vi "PH_Get6PInformation.set Sixpack Configuration.vi"(1 "Motor Type":T1, 2 "6P Axis Config Ref":refnum<vi>) -> (0 "6P Axis Config":T2 {"Axis Parameter"."Poslimit (6400)" step=1; "Ref Search Parameter"."DebouncingTime (22ms)" format="%.0x"; "I max (50%)" min=0.0 max=100.0})   [LabVIEW 2014, in "PH_Get6PInformation.lvlib"]
uses:
  PH_Get6PInformation.lvlib
  PH_Sixpack/PH_Sixpack.Axis Configuration.ctl
  instr.lib/SixPack/PackDLL/VmaxAmax.ctl
  instr.lib/SixPack/PackDLL/PeakCurrent.ctl
  instr.lib/SixPack/PackDLL/VStartVmin.ctl
  instr.lib/SixPack/PackDLL/Ref Search Parameter.ctl
  instr.lib/SixPack/PackDLL/Stopswitch Limits.ctl
  instr.lib/SixPack/PackDLL/Motor Parameter.ctl
  instr.lib/SixPack/PackDLL/MotorParameter_P5.ctl
  instr.lib/SixPack/PackDLL/MotorParameter_P6.ctl
  instr.lib/SixPack/PackDLL/Current Control.ctl
  instr.lib/SixPack/PackDLL/Current.ctl
  PH_Stepmotor_BaseClass/PH_Stepmotor_BaseClass.Motor Type.ctl
  PH_Sixpack/PH_Sixpack.lvlib
  instr.lib/SixPack/Sixpack - Driver.lvlib
  PH_Stepmotor_BaseClass/PH_Stepmotor_BaseClass.lvlib
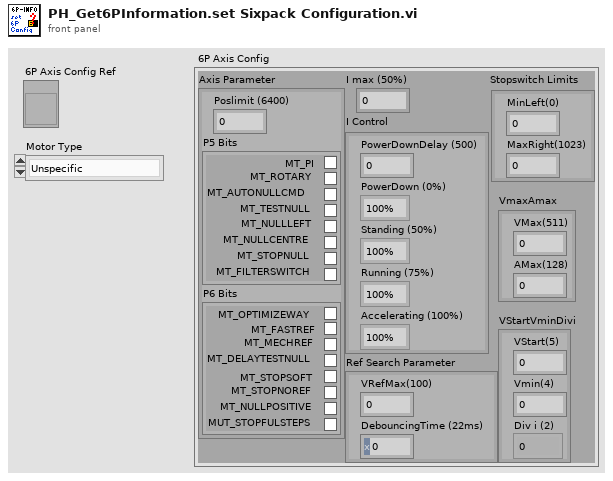
[diagram p1: front panel]
types:
  T1 = typedef "PH_Stepmotor_BaseClass.lvlib/PH_Stepmotor_BaseClass.Motor Type.ctl" = enum16{"Unspecific", "OWIS 49.120.2633", "OWIS 49.060.1033", "OWIS 43.040.2558", "Diamond Motion 2200 series", "OWIS 49.120.266B.MV6", "Calorimeter", "Linear Stage 1", "MICOS VT-80", "MICOS VT-80 S", "Standa Rotstage nt0.95A", "PUF RA 320.200", "PUF RA 800.200", "PUF RA 800.400", "PUF RA 400.50", "1324.nn.800.50", "1324.n9c.800.50", "1324.nn.320.200", "1324.nn.400.200", "1324.nn.800.200", "1324.nn.400.50", "1324.8c9c.800.50", "1324.8c9c.400.200"}
  T2 = typedef "PH_Sixpack.lvlib/PH_Sixpack.Axis Configuration.ctl" = cluster{"VmaxAmax":T3, "I max (50%)":T4, "VStartVminDivi":T5, "Ref Search Parameter":T6, "Stopswitch Limits":T7, "Axis Parameter":T8, "I Control":T11}
  T3 = typedef "Sixpack - Driver.lvlib/VmaxAmax.ctl" = cluster{"VMax(511)":u16, "AMax(128)":u16}
  T4 = typedef "Sixpack - Driver.lvlib/PeakCurrent.ctl" = dbl
  T5 = typedef "Sixpack - Driver.lvlib/VStartVmin.ctl" = cluster{"VStart(5)":u16, "Vmin(4)":u16, "Div i (2)":enum8{"0", "1", "2", "3"}}
  T6 = typedef "Sixpack - Driver.lvlib/Ref Search Parameter.ctl" = cluster{"VRefMax(100)":u16, "DebouncingTime (22ms)":u8}
  T7 = typedef "Sixpack - Driver.lvlib/Stopswitch Limits.ctl" = cluster{"MinLeft(0)":u16, "MaxRight(1023)":u16}
  T8 = typedef "Sixpack - Driver.lvlib/Motor Parameter.ctl" = cluster{"Poslimit (6400)":u32, "P5 Bits":T9, "P6 Bits":T10}
  T9 = typedef "Sixpack - Driver.lvlib/MotorParameter_P5.ctl" = cluster{"MT_PI":bool, "MT_ROTARY":bool, "MT_AUTONULLCMD":bool, "MT_TESTNULL":bool, "MT_NULLLEFT":bool, "MT_NULLCENTRE":bool, "MT_STOPNULL":bool, "MT_FILTERSWITCH":bool}
  T10 = typedef "Sixpack - Driver.lvlib/MotorParameter_P6.ctl" = cluster{"MT_OPTIMIZEWAY":bool, "MT_FASTREF":bool, "MT_MECHREF":bool, "MT_DELAYTESTNULL":bool, "MT_STOPSOFT":bool, "MT_STOPNOREF":bool, "MT_NULLPOSITIVE":bool, "MUT_STOPFULSTEPS":bool}
  T11 = typedef "Sixpack - Driver.lvlib/Current Control.ctl" = cluster{"PowerDownDelay (500)":u16, "PowerDown (0%)":T12, "Standing (50%)":T12, "Running (75%)":T12, "Accelerating (100%)":T12}
  T12 = typedef "Sixpack - Driver.lvlib/Current.ctl" = enum8{"100%", "75%", "50%", "38%", "25%", "19%", "13%", "9%", "0%"}
  T13 = enum8{"Enabled", "Disabled", "Disabled and Grayed Out"}
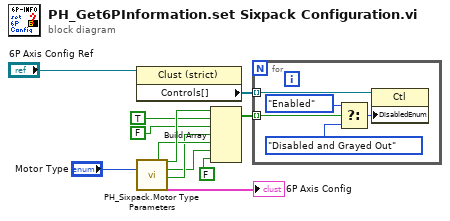
[diagram p0: block diagram]
diagram:
  n1 = property on="Property Node" class="Clust (strict)"(reference="6P Axis Config Ref") -> ("Controls[]"=w2:refnum<vi>[])  [unwired: 1 in, 2 out]
  n2 = call "PH_Sixpack.Motor Type Parameters.vi"("Motor Type"="Motor Type") -> ("Set Stopswitch Limits?"=w7:bool, "Set VmaxAmax"=w10:bool, "Set Axis Parameter"=w5:bool, "Set Ref Search Parameters"=w6:bool, "6P Axis Config"=→"6P Axis Config":T2)  [unwired: 17 in, 5 out]
  n3 = Build Array(w10, TRUE ("element"), FALSE ("element"), w6, w7, w5, FALSE ("element")) -> (w3:bool[])
  n4 = for {
    tunnel: w2 -> [w17] mode=indexing
    tunnel: w3 -> [w14] mode=indexing
    n5 = Select(t=T13."Enabled", s=w14, f=T13."Disabled and Grayed Out" ("Disabled")) -> (s? t:f=w15:T13)
    n6 = property class="Ctl"(reference=w17, "DisabledEnum"=w15) -> ()  [unwired: 1 in, 2 out]
  }
